vi "cRIO FPGA Read EEPROM_8 Slots.vi"(10 "Address":u16) -> (2 "Data Read":u8 format="%.0x")   [LabVIEW 2016]
uses:
  <vilib>/eio/EIONode/EIONode.xnode
  Instance           1 34Saved   cRIO FPGA - control eeprom .vi
  <vilib>/rvi/eio/common/nirviEmuTemplateMethod_errors.vi
panel:
  out "Data out":u8[](array[numeric])
  in  "Module":u16
  in  "Wakeup wait (ms)":u32=200
  in  "Stop":bool
  in  "Execute":bool
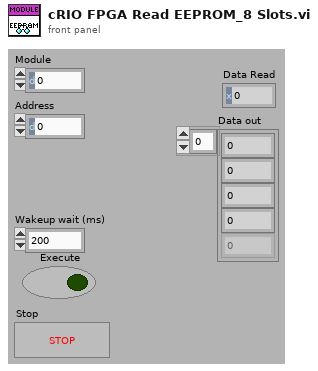
[diagram p1: front panel]
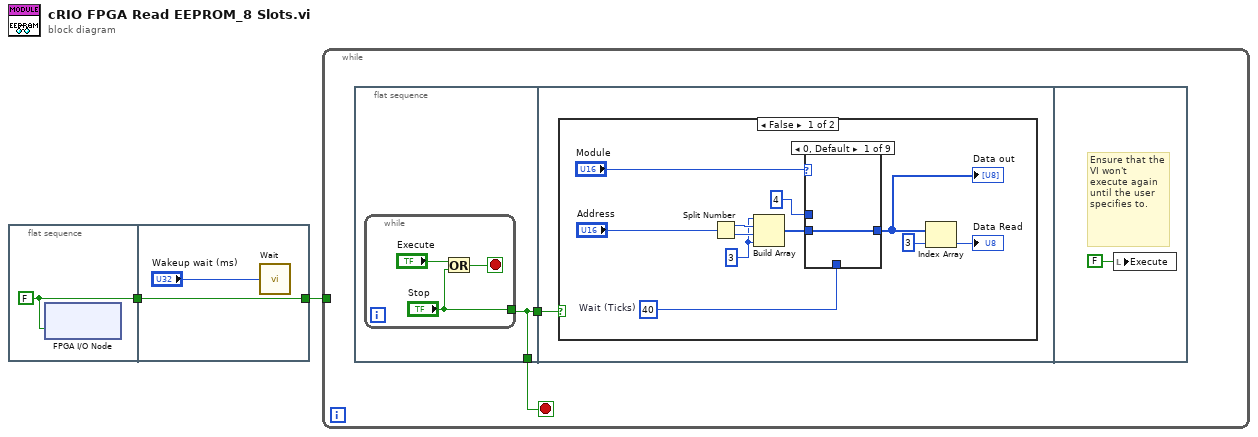
[diagram p0: block diagram]
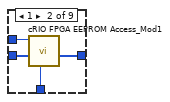
[diagram p2: hidden frame]
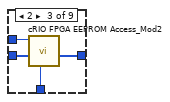
[diagram p3: hidden frame]
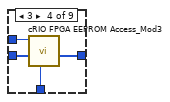
[diagram p4: hidden frame]
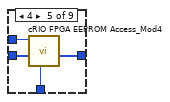
[diagram p5: hidden frame]
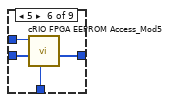
[diagram p6: hidden frame]
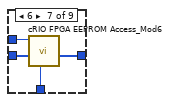
[diagram p7: hidden frame]
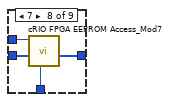
[diagram p8: hidden frame]
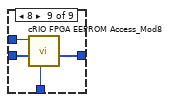
[diagram p9: hidden frame]
diagram:
  n1 = flat-sequence {
    tunnel: [w3] -> w2
    tunnel: [w4] -> w1
    tunnel: w2 -> [w4]
    frame #0 {
      w3 = FALSE ("Digital Out")
      n2 = xnode "FPGA I/O Node"("Sleep"=w3) -> ()  [unwired: 1 in, 1 out]
    }
    frame #1 {
      n3 = call "Wait"("Count(mSec)"="Wakeup wait (ms)") -> ()  [unwired: 1 out]
    }
  }
  n4 = while {
    tunnel: w1 -> [_]
    stop <- w6 stop-if-true
    n5 = flat-sequence {
      tunnel: [w8] -> w7
      tunnel: [w8] -> w6
      tunnel: w7 -> [w12]
      frame #0 {
        n6 = while {
          tunnel: ["Stop"] -> w8
          stop <- w11 stop-if-true
          n7 = Or(x="Execute", y="Stop") -> (x .or. y?=w11:bool)
        }
      }
      frame #1 {
        n8 = case shown="False" w12 {
          frame False {
            w18 = u8 3
            w21 = u8 40  # Wait (Ticks)
            n9 = Split Number(x="Address") -> (hi(x)=w20:u8, lo(x)=w19:u8)
            n10 = Build Array(w18, w20, w19, w18) -> (w17:u8[])
            n11 = case shown="0, Default" "Module" {
              tunnel: w21 -> [_ w28 w32 w36 w40 w44 w48 w52 w56]
              tunnel: w17 -> [w24 w27 w31 w35 w39 w43 w47 w51 w55]
              tunnel: u8 4 ("bytes") -> [_ w26 w30 w34 w38 w42 w46 w50 w54]
              tunnel: [w24 w25 w29 w33 w37 w41 w45 w49 w53] -> w15
              frame 0, Default {
              }
              frame 1 {
                n12 = call "cRIO FPGA EEPROM Access_Mod1.vi"("Wait (Ticks)"=w28, "Data in"=w27, "bytes"=w26) -> ("Data out"=w25:u8[])  [unwired: 8 in]
              }
              frame 2 {
                n13 = call "cRIO FPGA EEPROM Access_Mod2.vi"("Wait (Ticks)"=w32, "Data in"=w31, "bytes"=w30) -> ("Data out"=w29:u8[])  [unwired: 8 in]
              }
              frame 3 {
                n14 = call "cRIO FPGA EEPROM Access_Mod3.vi"("Wait (Ticks)"=w36, "Data in"=w35, "bytes"=w34) -> ("Data out"=w33:u8[])  [unwired: 8 in]
              }
              frame 4 {
                n15 = call "cRIO FPGA EEPROM Access_Mod4.vi"("Wait (Ticks)"=w40, "Data in"=w39, "bytes"=w38) -> ("Data out"=w37:u8[])  [unwired: 8 in]
              }
              frame 5 {
                n16 = call "cRIO FPGA EEPROM Access_Mod5.vi"("Wait (Ticks)"=w44, "Data in"=w43, "bytes"=w42) -> ("Data out"=w41:u8[])  [unwired: 8 in]
              }
              frame 6 {
                n17 = call "cRIO FPGA EEPROM Access_Mod6.vi"("Wait (Ticks)"=w48, "Data in"=w47, "bytes"=w46) -> ("Data out"=w45:u8[])  [unwired: 8 in]
              }
              frame 7 {
                n18 = call "cRIO FPGA EEPROM Access_Mod7.vi"("Wait (Ticks)"=w52, "Data in"=w51, "bytes"=w50) -> ("Data out"=w49:u8[])  [unwired: 8 in]
              }
              frame 8 {
                n19 = call "cRIO FPGA EEPROM Access_Mod8.vi"("Wait (Ticks)"=w56, "Data in"=w55, "bytes"=w54) -> ("Data out"=w53:u8[])  [unwired: 8 in]
              }
            }
            "Data out" <- w15
            n20 = Index Array(array=w15, index=3) -> (element=→"Data Read":u8)
          }
          frame True {
          }
        }
      }
      frame #2 {
        # "Ensure that the VI won't execute again until the user specifies to."
        n21 = local write "Execute"(FALSE) -> ()
      }
    }
  }
